vi "Scale.vi"(8 "error in (no error)":errorcluster, 11 "Sensor in":refnum<class "Sensor Config.lvclass">) -> (0 "error out":errorcluster, 2 "Sensor Scale":refnum<class "Scale Config.lvclass">, 3 "Sensor out":refnum<class "Sensor Config.lvclass">)   [LabVIEW 2020, in "VolatusConfig.lvlib" / "Sensor Config.lvclass"]
uses:
  Sensor Config.lvclass
  C:/dev/lv20CE/relink/lv-volatus/VolatusConfig/VolatusConfigElement/VolatusConfigElement.lvclass
  Scale/Scale Config.lvclass
  VolatusConfigElement/VolatusConfigElement.lvclass/VolatusConfigElement.ctl
  VolatusConfigElement/Element.vi
  Sensor Config.lvclass/Sensor Config.ctl
  VolatusConfigElement/VolatusConfigElement.lvclass
  C:/dev/lv20CE/relink/lv-volatus/VolatusConfig/Sensor/Sensor Config.lvclass
  C:/dev/lv20CE/relink/lv-volatus/VolatusConfig/Scale/Scale Config.lvclass
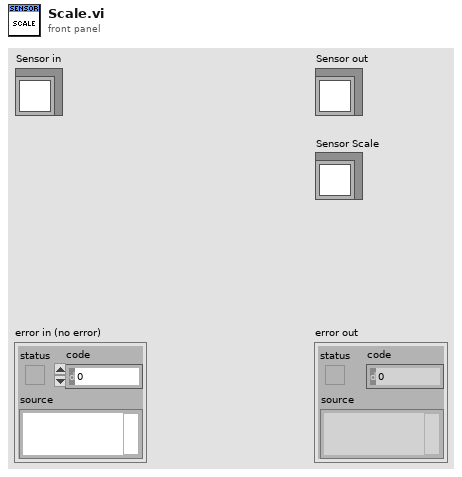
[diagram p1: front panel]
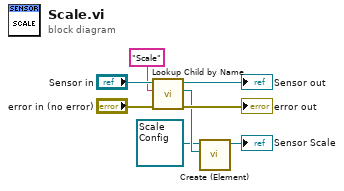
[diagram p0: block diagram]
diagram:
  n1 = call "Lookup Child by Name.vi"("error in (no error)"="error in (no error)", "Child Name"="Scale", "VolatusConfigElement in"="Sensor in") -> ("error out"=→"error out":errorcluster, "Child"=w4:refnum<class "Config Element.lvclass">, "VolatusConfigElement out"=→"Sensor out":refnum<class "Sensor Config.lvclass">)  [unwired: 5 in, 1 out]
  n2 = call "Create (Element).vi"("Element"=w4, "VolatusConfigElement in"=refnum<class "Scale Config.lvclass"> refnum ("VolatusConfig.lvlib:Scale")) -> ("VolatusConfigElement out"=→"Sensor Scale":refnum<class "Scale Config.lvclass">)  [unwired: 8 in, 1 out]
